vi "execute_initial_value_policy.vi"(8 "error in (no error)":errorcluster, 9 "Last Publish Time":timestamp, 10 "Last Topic Value":variant, 11 "ISubscriptionPolicy In":refnum<class "ISubscriptionPolicy.lvclass">) -> (0 "error out":errorcluster, 3 "ISubscriptionPolicy Out":refnum<class "ISubscriptionPolicy.lvclass">)   [LabVIEW 2015, in "IMediator.lvlib" / "ISubscriptionPolicy.lvclass"]
uses:
  ISubscriptionPolicy.lvclass
  ISubscriptionPolicy.lvclass/ISubscriptionPolicy.ctl
  ITransport/ITransport.lvclass
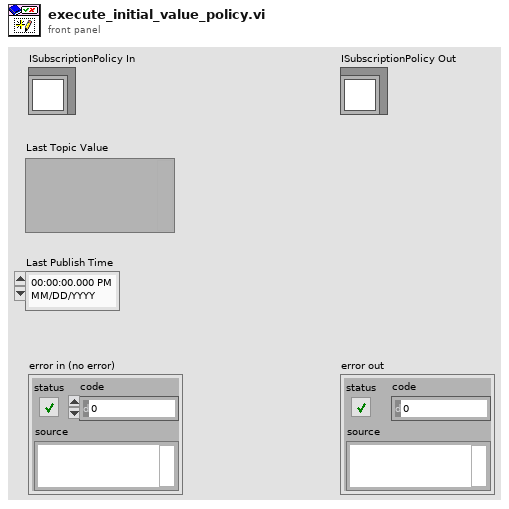
[diagram p1: front panel]
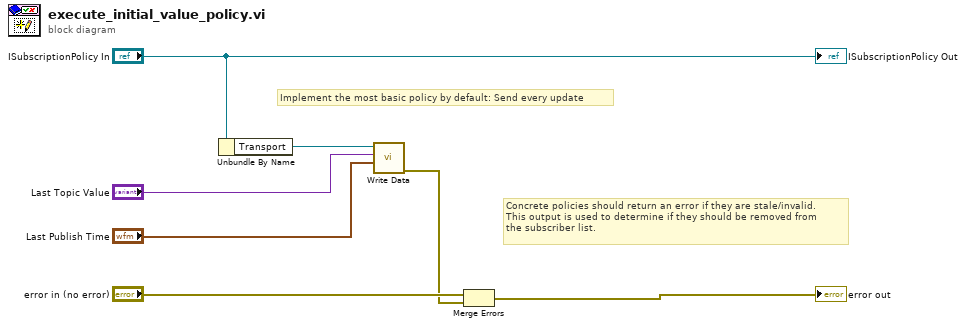
[diagram p0: block diagram]
diagram:
  # "Implement the most basic policy by default: Send every update"
  # "Concrete policies should return an error if they are stale/invalid.\nThis output is used to determine if they should be removed from\nthe subscriber list."
  n1 = Unbundle By Name("ISubscriptionPolicy In") -> ("Transport"=w5:refnum<class "ITransport.lvclass">)
  n2 = call-dynamic "Write Data.vi"("Publication Time"="Last Publish Time", "Value"="Last Topic Value", "ITransport in"=w5) -> ("error out"=w1:errorcluster)  [unwired: 7 in, 1 out]
  n3 = Merge Errors("error in (no error)", w1) -> (→"error out":errorcluster)
  "ISubscriptionPolicy Out" <- "ISubscriptionPolicy In"
